vi "Hardware config bundler-Boolean.vi"(7 "Keys setup.Boolean":T19, 8 "error in (no error)":errorcluster, 9 "Section name":string, 10 "Hardware Configuration I/P":T1={"Dev. PC"=FALSE, "Swap XY on stage"=FALSE, "No of AOD"=0, "MC Supported"=FALSE, "Axial MC"=FALSE, "Computer MAC address"="", "Externalise Triggers"=FALSE, "Trigger HW config"={"Available Device List"=0, "Device Address"=""}, "DAQmx Chan"={"Pockels AO"="", "Hard shutter AO"="", "PMT AOs"="", "Galvo AOs"="", "Power meter AI"=""}, "XYZ Stage Control Config"=enum."None", "XY stage available"=FALSE, "XY Comms Config Cluster"={"Name"="", "Device Address"="", "Port "=0, "Baudrate"=0, "Comms Type"=enum."GPIB-IEEE488"}, "Y stage available"=FALSE, "Y Comms Config Cluster"={"Name"="", "Device Address"="", "Port "=0, "Baudrate"=0, "Comms Type"=enum."GPIB-IEEE488"}, "Z stage available"=FALSE, "Z Comms Config Cluster "={"Name"="COM7", "Device Address"="", "Port "=0, "Baudrate"=0, "Comms Type"=enum."GPIB-IEEE488"}, "Encoder available"=FALSE, "Encoder"={"IP address"="224.0.1.103", "Port"=7000, "Wheel radius (cm)"=16.0, "Encoder Trigger"=""}, "VidRec available"=FALSE, "Cam VidRec"={"DO flag-Video record"="", "DO flag-Trial start"=""}, "Laser Power Control HW config"={"Laser Power Control"="", "Laser Power Modulation Control"=enum."NI"}, "Laser 1 available"=FALSE, "Laser 1 config cluster"={"COM port"="COM7", "Baud Rate"=0, "Type"=""}, "Prechirper 1 available"=FALSE, "Prechirper 1 config cluster"={"Type"="", "Baud Rate"=0, "COM port"="COM7"}, "Control system.FPGA available?"=FALSE, "Control Sys. HW config"={"Control system.FPGA Type"=enum."Virtex 5", "Control system.Network adapter name"="", "Control system.MAC address"="", "Control system.Ethernet Port"=0, "Control system.Ethernet Port Opened"=FALSE}, "DAQ FPGA HW Config"={"FGPA Ref"=refnum, "Target"="RIO0", "input card type"=enum."AC Card"}, "PMT Control Voltage Limits"={"Lower Limit"=0.0, "Upper Limit"=0.0}} {"Encoder"."Wheel radius (cm)" format="%#_13g"}, 11 "Refnum in":T18) -> (0 "error out":errorcluster, 2 "Hardware Configuration O/P":T1={"Dev. PC"=FALSE, "Swap XY on stage"=FALSE, "No of AOD"=0, "MC Supported"=FALSE, "Axial MC"=FALSE, "Computer MAC address"="", "Externalise Triggers"=FALSE, "Trigger HW config"={"Available Device List"=0, "Device Address"=""}, "DAQmx Chan"={"Pockels AO"="", "Hard shutter AO"="", "PMT AOs"="", "Galvo AOs"="", "Power meter AI"=""}, "XYZ Stage Control Config"=enum."None", "XY stage available"=FALSE, "XY Comms Config Cluster"={"Name"="", "Device Address"="", "Port "=0, "Baudrate"=0, "Comms Type"=enum."GPIB-IEEE488"}, "Y stage available"=FALSE, "Y Comms Config Cluster"={"Name"="", "Device Address"="", "Port "=0, "Baudrate"=0, "Comms Type"=enum."GPIB-IEEE488"}, "Z stage available"=FALSE, "Z Comms Config Cluster "={"Name"="COM7", "Device Address"="", "Port "=0, "Baudrate"=0, "Comms Type"=enum."GPIB-IEEE488"}, "Encoder available"=FALSE, "Encoder"={"IP address"="224.0.1.103", "Port"=7000, "Wheel radius (cm)"=16.0, "Encoder Trigger"=""}, "VidRec available"=FALSE, "Cam VidRec"={"DO flag-Video record"="", "DO flag-Trial start"=""}, "Laser Power Control HW config"={"Laser Power Control"="", "Laser Power Modulation Control"=enum."NI"}, "Laser 1 available"=FALSE, "Laser 1 config cluster"={"COM port"="COM7", "Baud Rate"=0, "Type"=""}, "Prechirper 1 available"=FALSE, "Prechirper 1 config cluster"={"Type"="", "Baud Rate"=0, "COM port"="COM7"}, "Control system.FPGA available?"=FALSE, "Control Sys. HW config"={"Control system.FPGA Type"=enum."Virtex 5", "Control system.Network adapter name"="", "Control system.MAC address"="", "Control system.Ethernet Port"=0, "Control system.Ethernet Port Opened"=FALSE}, "DAQ FPGA HW Config"={"FGPA Ref"=refnum, "Target"="RIO0", "input card type"=enum."AC Card"}, "PMT Control Voltage Limits"={"Lower Limit"=0.0, "Upper Limit"=0.0}} {"Encoder"."Wheel radius (cm)" format="%#_13g"}, 3 "Refnum out":T18)   [LabVIEW 2020]
uses:
  Typedefs/Ini file interface (Boolean).ctl
  <vilib>/Utility/config.llb/Config Data RefNum.ctl
  Typedefs/Hardware Configuration settings.ctl
  Typedefs/Triggers HW config.ctl
  Typedefs/DAQmx physical channels cluster.ctl
  Peripherals Control/XYZ Stage/Control/typedefs/XYZControlConfig.ctl
  Typedefs/Peripherals comms config cluster.ctl
  Typedefs/Comms Type.ctl
  Typedefs/Encoder config cluster.ctl
  Typedefs/Cam VidRec HW config setup cluster.ctl
  Typedefs/Laser Power Control HW config.ctl
  Typedefs/Laser 1 config cluster.ctl
  Typedefs/PreChirper 1 config cluster.ctl
  Typedefs/Control Sys HW config cluster.ctl
  Typedefs/DAQ FPGA HW config cluster.ctl
  RIG-SPECIFIC FILES/FPGA Refs/FPGA Ref.ctl
  <vilib>/userDefined/High Color/nirio_resource_hc.ctl
  Typedefs/FPGA input type AC-DC.ctl
  Typedefs/PMT Control Voltage limits.ctl
  <vilib>/Utility/config.llb/NI_LVConfig.lvlib
panel:
  # "(make , model etc)"
  # "(COM Port / IP Address / service address etc.)"
  # "(Port for ethernet / channel for BT)"
  # "(make , model etc)"
  # "(COM Port / IP Address / service address etc.)"
  # "(Port for ethernet / channel for BT)"
  # "(make , model etc)"
  # "(COM Port / IP Address / service address etc.)"
  # "(Port for ethernet / channel for BT)"
  # "(make , model etc)"
  # "(COM Port / IP Address / service address etc.)"
  # "(Port for ethernet / channel for BT)"
  # "(make , model etc)"
  # "(COM Port / IP Address / service address etc.)"
  # "(Port for ethernet / channel for BT)"
  # "(make , model etc)"
  # "(COM Port / IP Address / service address etc.)"
  # "(Port for ethernet / channel for BT)"
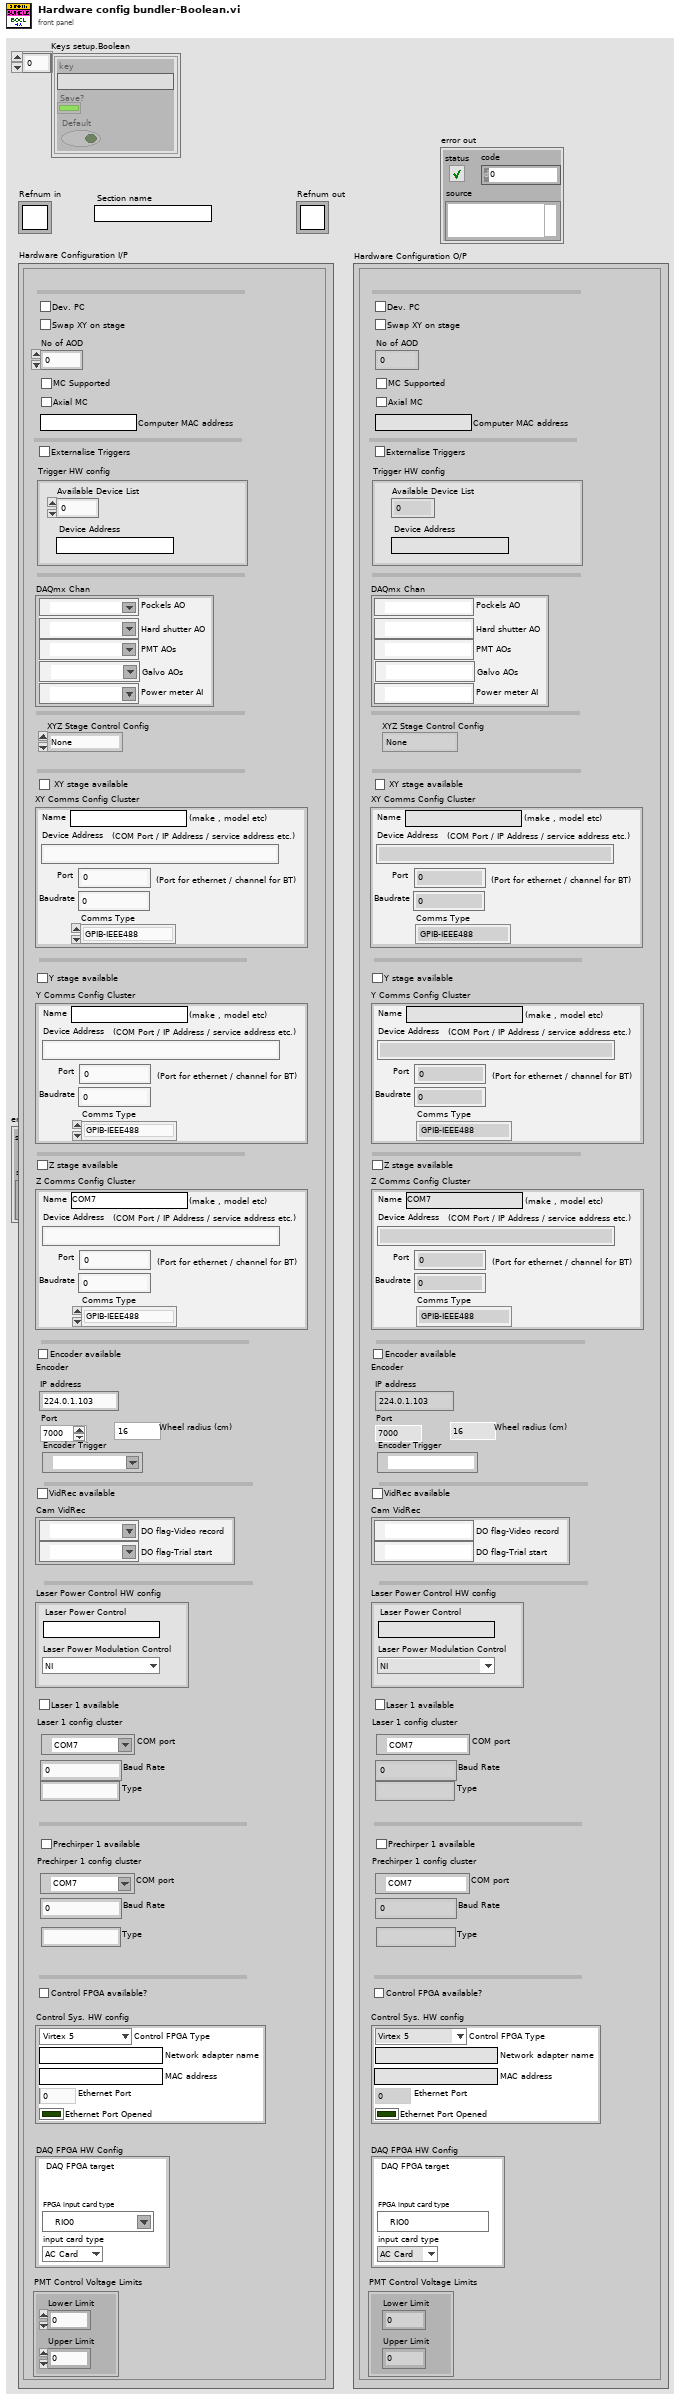
[diagram p1: front panel]
types:
  T1 = typedef "Hardware Configuration settings.ctl" = cluster{"Dev. PC":bool, "Swap XY on stage":bool, "No of AOD":u8, "MC Supported":bool, "Axial MC":bool, "Computer MAC address":string, "Externalise Triggers":bool, "Trigger HW config":T2, "DAQmx Chan":T3, "XYZ Stage Control Config":T4, "XY stage available":bool, "XY Comms Config Cluster":T5, "Y stage available":bool, "Y Comms Config Cluster":T5, "Z stage available":bool, "Z Comms Config Cluster ":T5, "Encoder available":bool, "Encoder":T7, "VidRec available":bool, "Cam VidRec":T8, "Laser Power Control HW config":T9, "Laser 1 available":bool, "Laser 1 config cluster":T10, "Prechirper 1 available":bool, "Prechirper 1 config cluster":T11, "Control system.FPGA available?":bool, "Control Sys. HW config":T12, "DAQ FPGA HW Config":T13, "PMT Control Voltage Limits":T17}
  T2 = typedef "Triggers HW config.ctl" = cluster{"Available Device List":i32, "Device Address":string}
  T3 = typedef "DAQmx physical channels cluster.ctl" = cluster{"Pockels AO":tag, "Hard shutter AO":tag, "PMT AOs":tag, "Galvo AOs":tag, "Power meter AI":tag}
  T4 = typedef "XYZControlConfig.ctl" = enum16{"None", "XYZ", "XY-Z", "X-Y-Z", "Z"}
  T5 = typedef "Peripherals comms config cluster.ctl" = cluster{"Name":string, "Device Address":string, "Port ":u16, "Baudrate":i32, "Comms Type":T6}
  T6 = typedef "Comms Type.ctl" = enum16{"GPIB-IEEE488", "Serial-RS232", "Serial-RS485", "Serial-RS422", "Serial-USB", "Ethernet-TCP/IP", "Ethernet-UDP"}
  T7 = typedef "Encoder config cluster.ctl" = cluster{"IP address":string, "Port":u16, "Wheel radius (cm)":dbl, "Encoder Trigger":tag}
  T8 = typedef "Cam VidRec HW config setup cluster.ctl" = cluster{"DO flag-Video record":tag, "DO flag-Trial start":tag}
  T9 = typedef "Laser Power Control HW config.ctl" = cluster{"Laser Power Control":string, "Laser Power Modulation Control":enum16{"NI", "FPGA"}}
  T10 = typedef "Laser 1 config cluster.ctl" = cluster{"COM port":refnum<visa-resource-name>, "Baud Rate":i32, "Type":string}
  T11 = typedef "PreChirper 1 config cluster.ctl" = cluster{"Type":string, "Baud Rate":i32, "COM port":refnum<visa-resource-name>}
  T12 = typedef "Control Sys HW config cluster.ctl" = cluster{"Control system.FPGA Type":enum16{"Virtex 5", "Virtex 7"}, "Control system.Network adapter name":string, "Control system.MAC address":string, "Control system.Ethernet Port":u32, "Control system.Ethernet Port Opened":bool}
  T13 = typedef "DAQ FPGA HW config cluster.ctl" = cluster{"FGPA Ref":T14, "Target":T15, "input card type":T16}
  T14 = typedef "FPGA Ref.ctl" = refnum<k20>
  T15 = typedef "nirio_resource_hc.ctl" = tag
  T16 = typedef "FPGA input type AC-DC.ctl" = enum16{"AC Card", "DC Card"}
  T17 = typedef "PMT Control Voltage limits.ctl" = cluster{"Lower Limit":dbl, "Upper Limit":dbl}
  T18 = typedef "NI_LVConfig.lvlib/Config Data RefNum.ctl" = refnum<k1>
  T19 = typedef "Ini file interface (Boolean).ctl" = cluster{"key":string, "Save?":bool, "Default":bool}[]
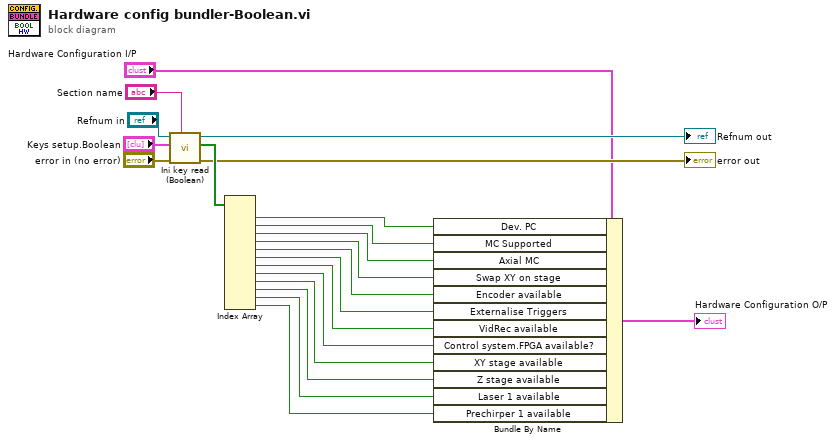
[diagram p0: block diagram]
diagram:
  n1 = call "Ini key read (Boolean).vi"("Section"="Section name", "error in (no error)"="error in (no error)", "Parameter names & setup"="Keys setup.Boolean", "Ini file refnum in"="Refnum in") -> ("error out"=→"error out":errorcluster, "Value read/used"=w16:bool[], "Ini file refnum out"=→"Refnum out":T18)  [unwired: 5 in]
  n2 = Index Array(array=w16) -> (element #1=w17:bool, element #2=w18:bool, element #3=w19:bool, element #4=w20:bool, element #5=w21:bool, element #6=w9:bool, element #7=w8:bool, element #8=w5:bool, element #9=w4:bool, element #10=w3:bool, element #11=w2:bool, element #12=w1:bool)  [unwired: 12 in]
  n3 = Bundle By Name(cluster="Hardware Configuration I/P", "Dev. PC"=w17, "MC Supported"=w18, "Axial MC"=w19, "Swap XY on stage"=w20, "Encoder available"=w21, "Externalise Triggers"=w9, "VidRec available"=w8, "Control system.FPGA available?"=w5, "XY stage available"=w4, "Z stage available"=w3, "Laser 1 available"=w2, "Prechirper 1 available"=w1) -> (→"Hardware Configuration O/P":T1)
